vi "Experiment header-bundle and save retrospective values.vi"(8 "error in (no error)":errorcluster) -> (0 "error out":errorcluster)   [LabVIEW 2017]
uses:
  Typedefs/Header file interface module functions enum.ctl
  Global Variables/General Globals.vi
  Typedefs/Header file type enum.ctl
panel:
  out "Parameter Value":dbl[](array[numeric])
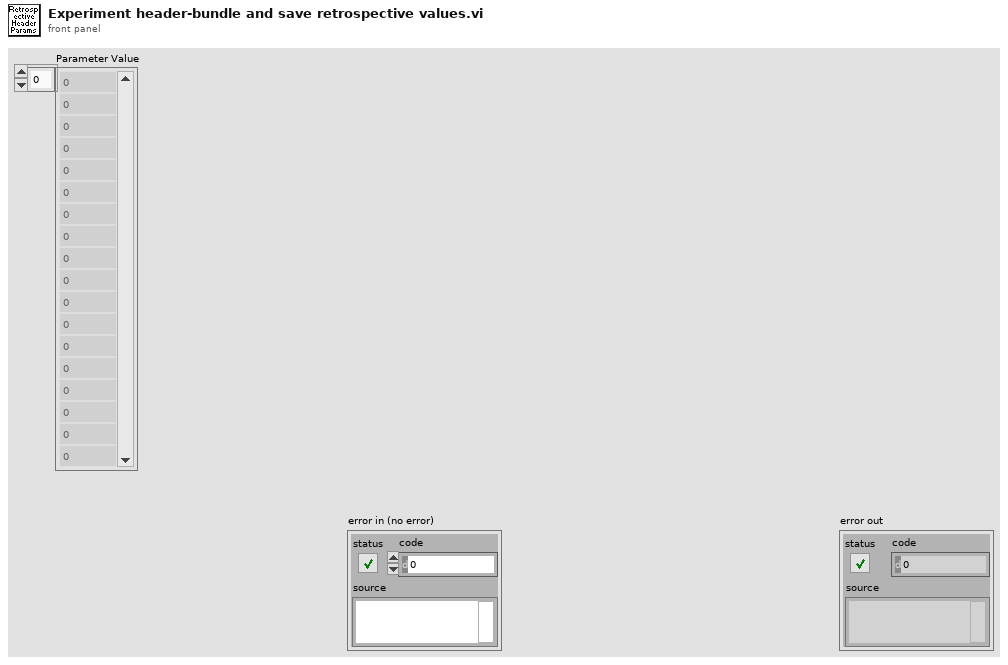
[diagram p1: front panel]
types:
  T1 = typedef "Header file type enum.ctl" = enum16{"All parameters", "Params for funct acq w ROI or mscn", "Params for funct acq w rectangles", "Live imaging header parameters", "AOL Parameters"}
  T2 = typedef "Header file interface module functions enum.ctl" = enum16{"Load experiment header file", "Save experiment header file", "Clear stored values", "Read stored values", "Update specific value in memory", "Update all values in memory"}
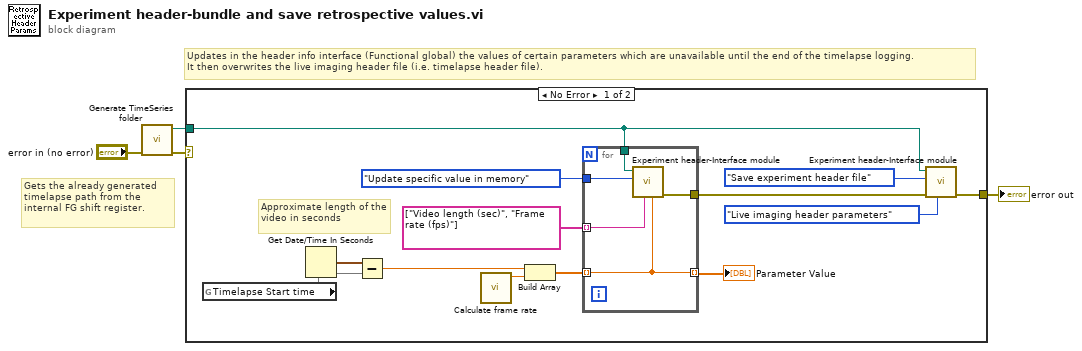
[diagram p0: block diagram]
diagram:
  # "Gets the already generated timelapse path from the internal FG shift register."
  # "Updates in the header info interface (Functional global) the values of certain parameters which are unavailable until the end of the timelapse logging. \nIt then overwrites the live imaging header file (i.e. timelapse header file)."
  n1 = call "Generate TimeSeries folder.vi"("error in (no error)"="error in (no error)") -> ("error out"=w3:errorcluster, "Timelapse folder path"=w1:path)  [unwired: 9 in]
  n2 = case shown="No Error" w3 {
    selector: w3 -> [_ w23]
    tunnel: [w17 w23] -> w4
    tunnel: w1 -> [w6 _]
    frame No Error {
      # "Approximate length of the video in seconds"
      n3 = global read "General Globals.vi" "Timelapse Start time"() -> (w10)
      n4 = Get Date/Time In Seconds() -> (seconds since 1Jan1904=w11:timestamp)
      n5 = Subtract(x=w11, y=w10) -> (x-y=w9:dbl)
      n6 = call "Calculate frame rate.vi"() -> ("Frame rate (fps)"=w5:dbl)  [unwired: 11 in]
      n7 = Build Array(w9, w5) -> (w13:dbl[])
      n8 = for {
        tunnel: string[] ["Video length (sec)", "Frame rate (fps)"] -> [w19] mode=indexing
        tunnel: w13 -> [w22] mode=indexing
        tunnel: [w22] -> w16 mode=indexing
        tunnel: [w21] -> w14
        tunnel: w6 -> [w20]
        tunnel: Header_file_interface_module_functions_enum."Update specific value in memory" ("Function") -> [w18]
        n9 = call "Experiment header-Interface module.vi"("New Value"=w22, "Name of parameter to update"=w19, "Function"=w18, "Experiment data folder path"=w20) -> ("error out"=w21:errorcluster)  [unwired: 6 in, 1 out]
      }
      "Parameter Value" <- w16
      n10 = call "Experiment header-Interface module.vi"("Header file type"=Header_file_type_enum."Live imaging header parameters", "error in (no error)"=w14, "Function"=Header_file_interface_module_functions_enum."Save experiment header file", "Experiment data folder path"=w6) -> ("error out"=w17:errorcluster)  [unwired: 6 in, 1 out]
    }
    frame Error {
    }
  }
  "error out" <- w4
